vi "Chocprocesssystem.vi"() -> ()   [LabVIEW 2021]
uses:
  <vilib>/Utility/file.llb/Write Delimited Spreadsheet (string).vi
panel:
  out "DISPLAY":T1
  out "CURRENT PROCESS":string
  out "TOTAL EVENTS":i32
  out "TIME":string
  out "DATE":string
  out "SUGAR":dbl
  out "MOULDING":bool
  in  "EMERGENCY":bool
  out "PACK":dbl(slide)
  out "Vanilla":u8(slide)
  out "Milk/Milk Powder":u8(slide)
  out "Cocoa Liquor":u8(slide)
  out "Blend Type":string
  out "Sugar":bool
  out "Cocoa butter":bool
  out "Conve 2":dbl(slide) scale=0.0..10.0
  out "MIXING 2":bool
  out "MIXING":bool
  out "GRINDING":bool
  out "SPEED":dbl
  out "BLOWER":bool
  out "P1 STATUS":bool
  out "Conve":dbl(slide) scale=0.0..10.0
  out "Roast":dbl(slide) scale=0.0..100.0
  # "CHOCOLATE PROCESSING SYSTEM"
  # "Phase-I"
  # "Control Center"
  # "WAREHOUSE"
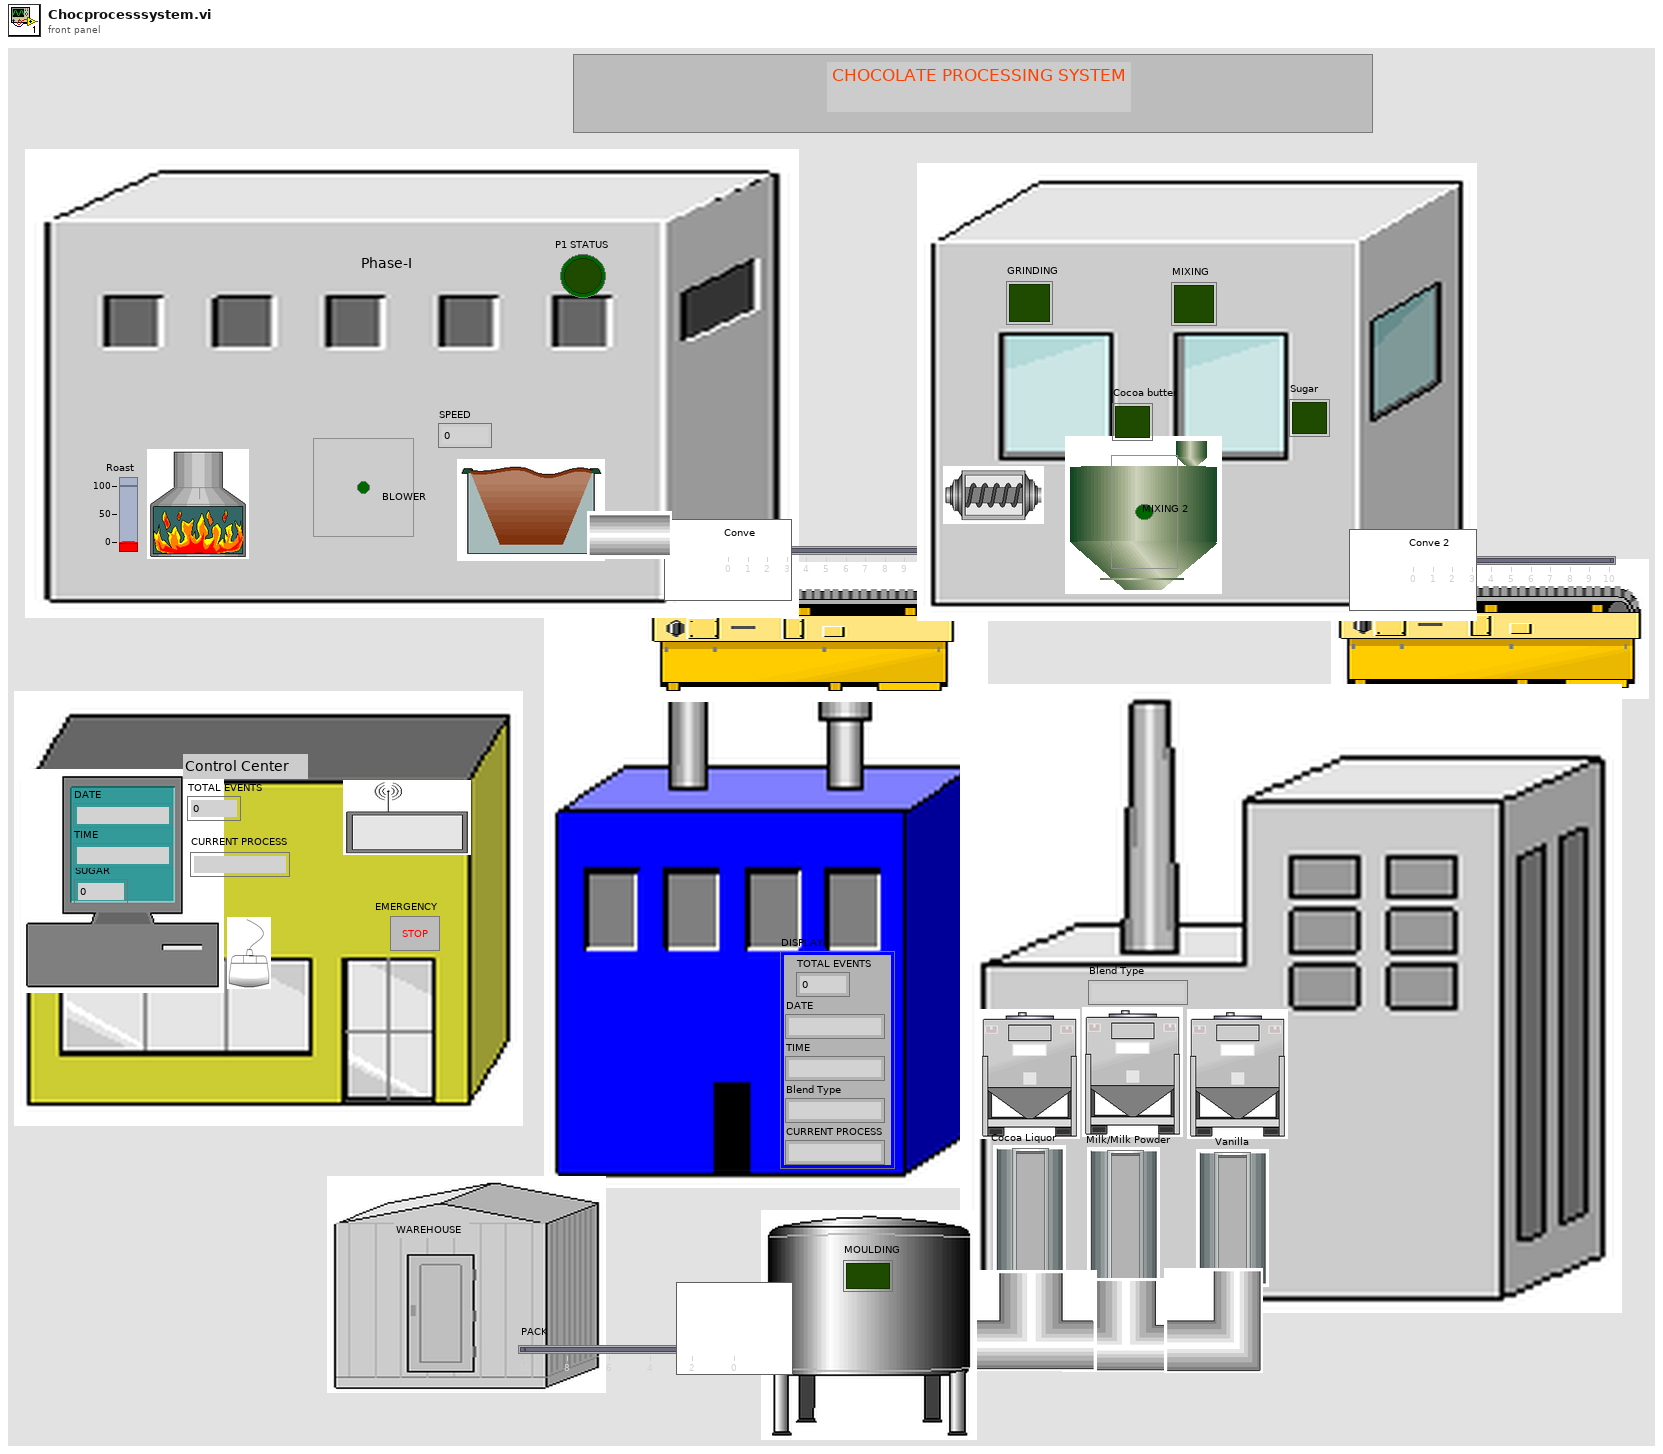
[diagram p1: front panel]
types:
  T1 = cluster{"TOTAL EVENTS":i32, "DATE":string, "TIME":string, "Blend Type":string, "CURRENT PROCESS":string}
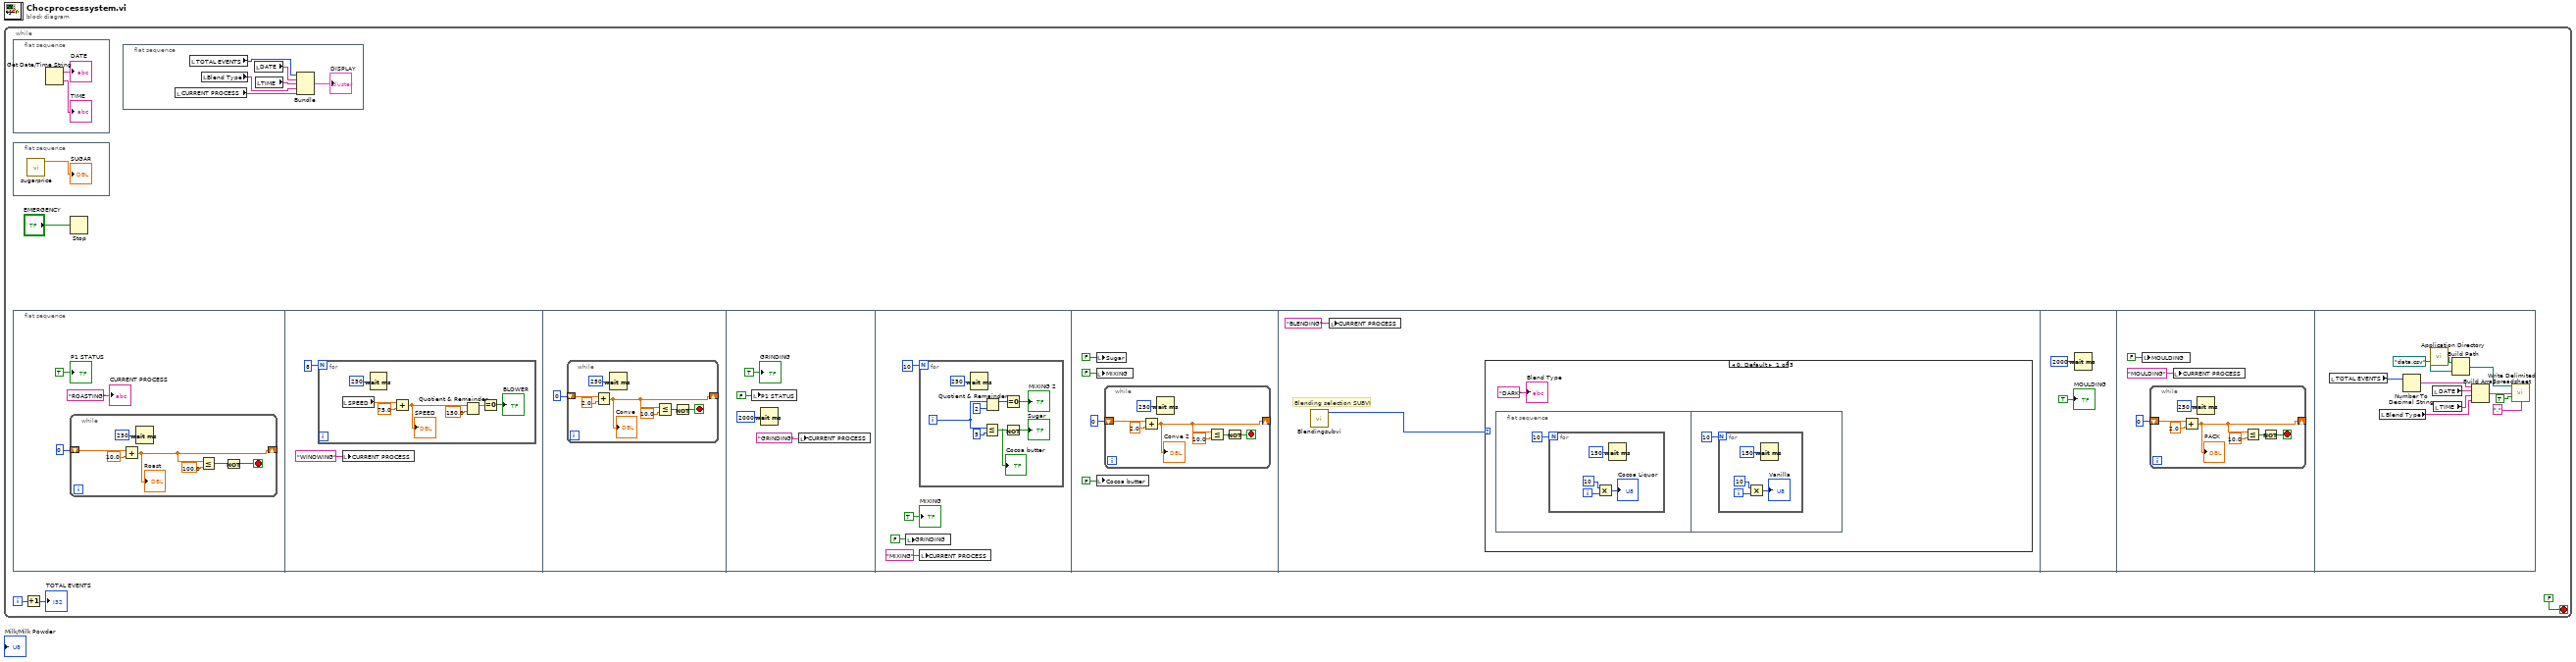
[diagram p0: block diagram]
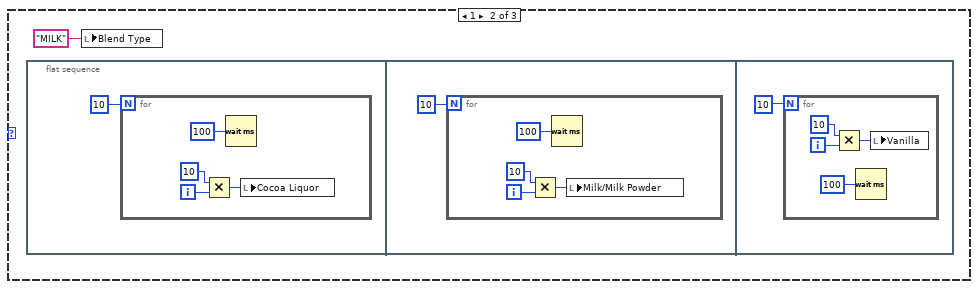
[diagram p2: hidden frame]
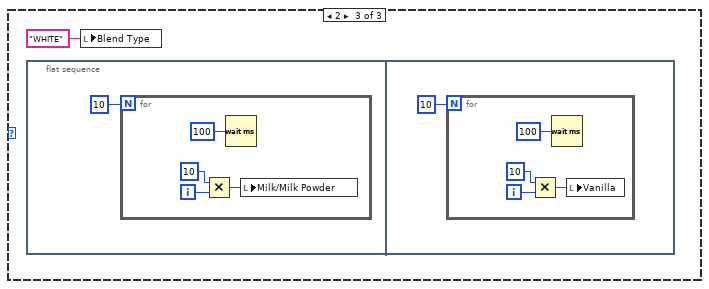
[diagram p3: hidden frame]
diagram:
  n1 = while {
    i -> [w2]
    stop <- FALSE stop-if-true
    n2 = flat-sequence {
      frame #0 {
        n3 = Get Date/Time String() -> (date string=→"DATE":string, time string=→"TIME":string)  [unwired: 3 in]
      }
    }
    n4 = flat-sequence {
      frame #0 {
        n5 = call "sugarprice.vi"() -> ("Numeric"=→"SUGAR":dbl)  [unwired: 11 in]
      }
    }
    n6 = flat-sequence {
      frame #0 {
        n7 = while {
          shift-right: [w21] -> _
          shift-left: 0 -> [w22]
          stop <- w18 stop-if-true
          n8 = Add(x=w22, y=10.0) -> (x+y=w21:dbl)
          "Roast" <- w21
          n9 = Wait (ms)(milliseconds to wait=u32 250) -> ()  [unwired: 1 out]
          n10 = Less Or Equal?(x=w21, y=100.0) -> (x <= y?=w17:bool)
          n11 = Not(x=w17) -> (.not. x?=w18:bool)
        }
        "P1 STATUS" <- TRUE ("P1 STATUS")
        "CURRENT PROCESS" <- "ROASTING"
      }
      frame #1 {
        n12 = for {
          N: 8 -> [_]
          n13 = local read "SPEED"() -> (w32:dbl)
          n14 = Wait (ms)(milliseconds to wait=u32 250) -> ()  [unwired: 1 out]
          n15 = Add(x=w32, y=75.0) -> (x+y=w29:dbl)
          "SPEED" <- w29
          n16 = Quotient & Remainder(x=w29, y=150.0) -> (x-y*floor(x/y)=w28:dbl)  [unwired: 1 out]
          n17 = Equal To 0?(x=w28) -> (x = 0?=→"BLOWER":bool)
        }
        n18 = local write "CURRENT PROCESS"("WINOWING" ("CURRENT PROCESS")) -> ()
      }
      frame #2 {
        n19 = while {
          shift-right: [w34] -> _
          shift-left: 0 -> [w39]
          stop <- w37 stop-if-true
          n20 = Add(x=w39, y=2.0) -> (x+y=w34:dbl)
          "Conve" <- w34
          n21 = Wait (ms)(milliseconds to wait=u32 250) -> ()  [unwired: 1 out]
          n22 = Less Or Equal?(x=w34, y=10.0) -> (x <= y?=w36:bool)
          n23 = Not(x=w36) -> (.not. x?=w37:bool)
        }
      }
      frame #3 {
        n24 = local write "P1 STATUS"(FALSE ("P1 STATUS")) -> ()
        n25 = Wait (ms)(milliseconds to wait=u32 2000) -> ()  [unwired: 1 out]
        n26 = local write "CURRENT PROCESS"("GRINDING" ("CURRENT PROCESS")) -> ()
        "GRINDING" <- TRUE ("GRINDING")
      }
      frame #4 {
        n27 = local write "GRINDING"(FALSE ("GRINDING")) -> ()
        n28 = for {
          N: 10 -> [_]
          i -> [w52]
          n29 = Wait (ms)(milliseconds to wait=u32 250) -> ()  [unwired: 1 out]
          n30 = Less Or Equal?(x=w52, y=5) -> (x <= y?=w49:bool)
          "Cocoa butter" <- w49
          n31 = Quotient & Remainder(x=w52, y=2) -> (x-y*floor(x/y)=w55:i32)  [unwired: 1 out]
          n32 = Equal To 0?(x=w55) -> (x = 0?=→"MIXING 2":bool)
          n33 = Not(x=w49) -> (.not. x?=→"Sugar":bool)
        }
        n34 = local write "CURRENT PROCESS"("MIXING" ("CURRENT PROCESS")) -> ()
        "MIXING" <- TRUE ("MIXING")
      }
      frame #5 {
        n35 = local write "Sugar"(FALSE ("Sugar")) -> ()
        n36 = local write "MIXING"(FALSE ("MIXING")) -> ()
        n37 = local write "Cocoa butter"(FALSE ("Cocoa butter")) -> ()
        n38 = while {
          shift-right: [w61] -> _
          shift-left: 0 -> [w66]
          stop <- w64 stop-if-true
          n39 = Add(x=w66, y=2.0) -> (x+y=w61:dbl)
          "Conve 2" <- w61
          n40 = Wait (ms)(milliseconds to wait=u32 250) -> ()  [unwired: 1 out]
          n41 = Less Or Equal?(x=w61, y=10.0) -> (x <= y?=w63:bool)
          n42 = Not(x=w63) -> (.not. x?=w64:bool)
        }
      }
      frame #6 {
        # "Blending selection SUBVI"
        n43 = call "Blendingsubvi.vi"() -> ("index of element"=w69:i32)  [unwired: 11 in]
        n44 = local write "CURRENT PROCESS"("BLENDING" ("CURRENT PROCESS")) -> ()
        n45 = case shown="0, Default" w69 {
          frame 0, Default {
            n46 = flat-sequence {
              frame #0 {
                n47 = for {
                  N: 10 -> [_]
                  i -> [w75]
                  n48 = Multiply(x=10, y=w75) -> (x*y=→"Cocoa Liquor":i32)
                  n49 = Wait (ms)(milliseconds to wait=u32 150) -> ()  [unwired: 1 out]
                }
              }
              frame #1 {
                n50 = for {
                  N: 10 -> [_]
                  i -> [w80]
                  n51 = Multiply(x=10, y=w80) -> (x*y=→"Vanilla":i32)
                  n52 = Wait (ms)(milliseconds to wait=u32 150) -> ()  [unwired: 1 out]
                }
              }
            }
            "Blend Type" <- "DARK" ("Blend Type")
          }
          frame 1 {
            n53 = flat-sequence {
              frame #0 {
                n54 = for {
                  N: 10 -> [_]
                  i -> [w86]
                  n55 = Multiply(x=10, y=w86) -> (x*y=w83:i32)
                  n56 = Wait (ms)(milliseconds to wait=u32 100) -> ()  [unwired: 1 out]
                  n57 = local write "Cocoa Liquor"(w83) -> ()
                }
              }
              frame #1 {
                n58 = for {
                  N: 10 -> [_]
                  i -> [w90]
                  n59 = Multiply(x=10, y=w90) -> (x*y=w88:i32)
                  n60 = Wait (ms)(milliseconds to wait=u32 100) -> ()  [unwired: 1 out]
                  n61 = local write "Milk/Milk Powder"(w88) -> ()
                }
              }
              frame #2 {
                n62 = for {
                  N: 10 -> [_]
                  i -> [w95]
                  n63 = Multiply(x=10, y=w95) -> (x*y=w93:i32)
                  n64 = Wait (ms)(milliseconds to wait=u32 100) -> ()  [unwired: 1 out]
                  n65 = local write "Vanilla"(w93) -> ()
                }
              }
            }
            n66 = local write "Blend Type"("MILK" ("Blend Type")) -> ()
          }
          frame 2 {
            n67 = flat-sequence {
              frame #0 {
                n68 = for {
                  N: 10 -> [_]
                  i -> [w102]
                  n69 = Multiply(x=10, y=w102) -> (x*y=w99:i32)
                  n70 = Wait (ms)(milliseconds to wait=u32 100) -> ()  [unwired: 1 out]
                  n71 = local write "Milk/Milk Powder"(w99) -> ()
                }
              }
              frame #1 {
                n72 = for {
                  N: 10 -> [_]
                  i -> [w106]
                  n73 = Multiply(x=10, y=w106) -> (x*y=w104:i32)
                  n74 = Wait (ms)(milliseconds to wait=u32 100) -> ()  [unwired: 1 out]
                  n75 = local write "Vanilla"(w104) -> ()
                }
              }
            }
            n76 = local write "Blend Type"("WHITE" ("Blend Type")) -> ()
          }
        }
      }
      frame #7 {
        n77 = Wait (ms)(milliseconds to wait=u32 2000) -> ()  [unwired: 1 out]
        "MOULDING" <- TRUE ("MOULDING")
      }
      frame #8 {
        n78 = local write "MOULDING"(FALSE ("MOULDING")) -> ()
        n79 = while {
          shift-right: [w113] -> _
          shift-left: 0 -> [w118]
          stop <- w116 stop-if-true
          n80 = Add(x=w118, y=2.0) -> (x+y=w113:dbl)
          "PACK" <- w113
          n81 = Wait (ms)(milliseconds to wait=u32 250) -> ()  [unwired: 1 out]
          n82 = Less Or Equal?(x=w113, y=10.0) -> (x <= y?=w115:bool)
          n83 = Not(x=w115) -> (.not. x?=w116:bool)
        }
        n84 = local write "CURRENT PROCESS"("MOULDING" ("CURRENT PROCESS")) -> ()
      }
      frame #9 {
        n85 = local read "TOTAL EVENTS"() -> (w124:i32)
        n86 = local read "Blend Type"() -> (w128:string)
        n87 = Number To Decimal String(number=w124) -> (decimal integer string=w127:string)  [unwired: 1 in]
        n88 = call <vilib>:"Application Directory.vi"() -> ("Application Directory"=w123:path)
        n89 = local read "DATE"() -> (w130:string)
        n90 = local read "TIME"() -> (w129:string)
        n91 = Build Path(base path=w123, name or relative path=path "data.csv") -> (appended path=w121:path)
        n92 = Build Array(w127, w130, w129, w128) -> (w126:string[])
        n93 = call-poly <vilib>:"Write Delimited Spreadsheet.vi"("file path (dialog if empty)"=w121, "1D data"=w126, "append to file? (new file:F)"=TRUE, "delimiter (\\t)"="," ("delimiter (\\t)")) -> ()  [unwired: 10 in, 2 out]
      }
    }
    n94 = Increment(x=w2) -> (x+1=→"TOTAL EVENTS":i32)
    n95 = Stop(stop? (T)="EMERGENCY") -> ()
    n96 = flat-sequence {
      frame #0 {
        n97 = local read "CURRENT PROCESS"() -> (w6:string)
        n98 = local read "TOTAL EVENTS"() -> (w8:i32)
        n99 = local read "Blend Type"() -> (w7:string)
        n100 = local read "DATE"() -> (w10:string)
        n101 = local read "TIME"() -> (w9:string)
        n102 = Bundle("TOTAL EVENTS"=w8, "DATE"=w10, "TIME"=w9, "Blend Type"=w7, "CURRENT PROCESS"=w6) -> (→"DISPLAY":T1)  [unwired: 1 in]
      }
    }
  }
